vi "NewCore.vi"(8 "error in (no error)":errorcluster, 10 "ParamsArray":variant[](array[variant]), 11 "EnchantedRoom":refnum<class "EnchantedRoom.lvclass">) -> (0 "error out":errorcluster, 3 "EnchantedRoom":refnum<class "EnchantedRoom.lvclass">)   [LabVIEW 2020, in "EnchantedRoom.lvclass"]
uses:
  EnchantedRoom.lvclass
  Private/TypeDef/privateData.ctl
  Spell/Spell.lvclass
  TypeDef/EnchantedRoomParams.ctl
  EnchantedRoom.lvclass/EnchantedRoom.ctl
  Room/Room.lvclass
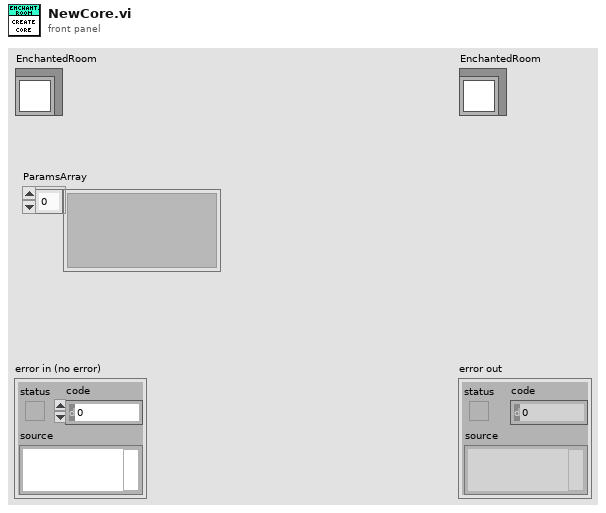
[diagram p1: front panel]
types:
  T1 = typedef "EnchantedRoom.lvclass/EnchantedRoomParams.ctl" = cluster{"Spell":refnum<class "Spell.lvclass">}
  T2 = typedef "EnchantedRoom.lvclass/privateData.ctl" = cluster{"Spell":refnum<class "Spell.lvclass">}
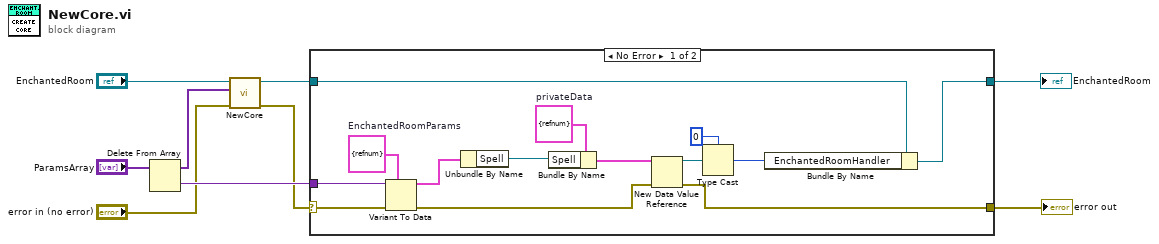
[diagram p0: block diagram]
diagram:
  n1 = Delete From Array(array="ParamsArray") -> (deleted portion=w4:variant, array with subset deleted=w3:variant[])  [unwired: 2 in]
  n2 = call-parent "NewCore.vi"("error in (no error)"="error in (no error)", "ParamsArray"=w3, "Room"="EnchantedRoom") -> ("error out"=w2:errorcluster, "Room"=w9:refnum<class "EnchantedRoom.lvclass">)  [unwired: 7 in]
  n3 = case shown="No Error" w2 {
    selector: w2 -> [w12 w25]
    tunnel: [w16 w25] -> w7
    tunnel: [w18 w24] -> w8
    tunnel: w9 -> [w17 w24]
    tunnel: w4 -> [w10 _]
    frame No Error {
      w14 = T1 {"Spell"=refnum}  # EnchantedRoomParams
      w20 = T2 {"Spell"=refnum}  # privateData
      n4 = Variant To Data(error in=w12, type=w14, Variant=w10) -> (data=w13:T1, error out=w11:errorcluster)
      n5 = Unbundle By Name(w13) -> ("Spell"=w15:refnum<class "Spell.lvclass">)
      n6 = Bundle By Name(cluster=w20, "Spell"=w15) -> (w19:T2)
      n7 = New Data Value Reference(data value=w19, error in=w11) -> (data value reference=w23:refnum<data-value>, error out=w16:errorcluster)
      n8 = Type Cast(type=u32 0, x=w23) -> (*(type *) &x=w21:u32)
      n9 = Bundle By Name(cluster=w17, "EnchantedRoomHandler"=w21) -> (w18:refnum<class "EnchantedRoom.lvclass">)
    }
    frame Error {
    }
  }
  "error out" <- w7
  "EnchantedRoom" <- w8
